vi "Define HVHST Test Array.vi"(9 "end":dbl=31.0, 11 "start":dbl=27.0) -> (3 "Ramp Pattern":dbl[](array[numeric]))   [LabVIEW 2013]
uses:
  <vilib>/Analysis/1siggen.llb/Ramp Pattern by Delta.vi
  <vilib>/Analysis/NI_AALBase.lvlib
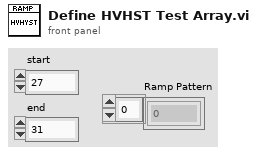
[diagram p1: front panel]
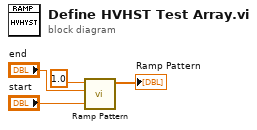
[diagram p0: block diagram]
diagram:
  n1 = call-poly <vilib>:"Ramp Pattern.vi"("start"="start", "end"="end", "delta"=1.0) -> ("Ramp Pattern"=→"Ramp Pattern":dbl[])  [unwired: 6 in, 2 out]
